vi "CtrlFindHandler.vi"(3 "Type":T1=enum."Value Change", 4 "Ctrl":refnum<vi>, 5 "Structure":refnum<vi>) -> (0 "Index":i32, 1 "Frame":i32, 2 "Diagram":refnum<vi>)   [LabVIEW 2014]
uses:
  <vilib>/event_ctls.llb/lveventtype.ctl
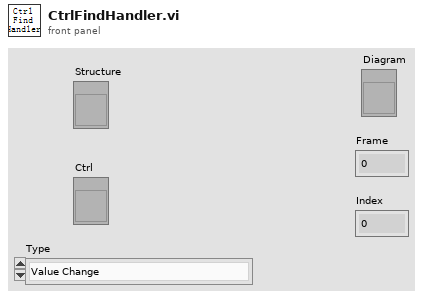
[diagram p1: front panel]
types:
  T1 = typedef "lveventtype.ctl" = enum32{"Null", "Timeout", "Annotation Menu Selection", "Annotation Menu Selection?", "App Instance Close", "App Instance Close?", "Autoscale Range Change", "Bookmark Info Change", "Cell Edit", "Cell Edit?", "Cursor Grab", "Cursor Grab?", "Cursor Menu Selection", "Cursor Menu Selection?", "Cursor Move", "Cursor Release", "Data Change", "Direction Change", "Display State Change", "Drag Ended", "Drag Enter", "Drag Leave", "Drag Over", "Drag Source Update", "Drag Starting", "Drag Starting?", "Drop", "Exec State Change", "Key Down", "Key Down?", "Key Repeat", "Key Repeat?", "Key Up", "Listbox Double Click", "Menu Activation?", "Menu Selection (App)", "Menu Selection? (App)", "Menu Selection (User)", "Mouse Down", "Mouse Down?", "Mouse Enter", "Mouse Leave", "Mouse Move", "Mouse Up", "Mouse Wheel", "NI Security User Change (App)", "Pane Size", "Panel Close", "Panel Close?", "Panel Resize", "Plot Attribute Change", "Scale Range Change", "Shortcut Menu Activation?", "Shortcut Menu Selection (App)", "Shortcut Menu Selection? (App)", "Shortcut Menu Selection (User)", "Tree Double Click", "Tree Drag", "Tree Drag?", "Tree Drop", "Tree Drop?", "Tree Item Close", "Tree Item Close?", "Tree Item Open", "Tree Item Open?", "User Event", "Value Change"}
  T2 = cluster{"Event Type":T1, "Reference":refnum<vi>, "Limit (-1=none)":i32, "Lock Panel?":bool}[]
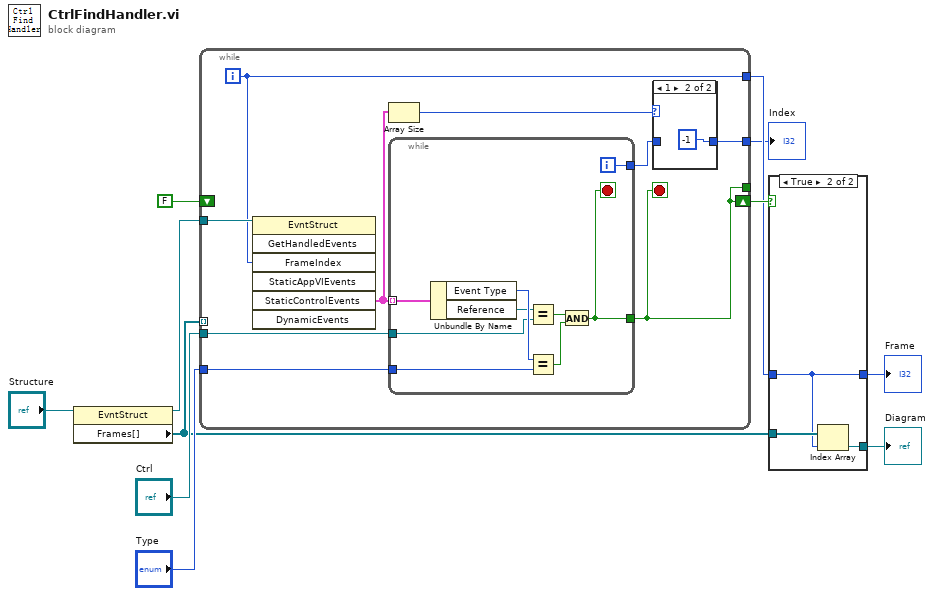
[diagram p0: block diagram]
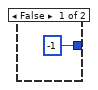
[diagram p2: hidden frame]
diagram:
  n1 = property class="EvntStruct"(reference="Structure") -> (reference out=w10:refnum<vi>, "Frames[]"=w2:refnum<vi>[])  [unwired: 1 in, 1 out]
  n2 = while {
    tunnel: "Type" -> [w20]
    tunnel: "Ctrl" -> [w19]
    tunnel: w10 -> [w18]
    tunnel: [w17] -> w5
    shift-right: [w16] -> w6
    shift-left: FALSE -> [_]
    tunnel: w2 -> [_] mode=indexing
    tunnel: [w16] -> _
    tunnel: [w12] -> w3
    i -> [w17]
    stop <- w16 stop-if-true
    n3 = invoke class="EvntStruct" method="GetHandledEvents"(reference=w18, "FrameIndex"=w17) -> ("StaticControlEvents"=w15:T2)  [unwired: 5 in, 6 out]
    n4 = Array Size(array=w15) -> (size(s)=w14:i32)
    n5 = while {
      tunnel: w15 -> [w31] mode=indexing
      tunnel: w20 -> [w29]
      tunnel: w19 -> [w27]
      tunnel: [w24] -> w16
      tunnel: [w23] -> w13
      i -> [w23]
      stop <- w24 stop-if-true
      n6 = Unbundle By Name(w31) -> ("Event Type"=w30:T1, "Reference"=w28:refnum<vi>)
      n7 = Equal?(x=w28, y=w27) -> (x = y?=w26:bool)
      n8 = Equal?(x=w30, y=w29) -> (x = y?=w25:bool)
      n9 = And(x=w26, y=w25) -> (x .and. y?=w24:bool)
    }
    n10 = case shown="1" w14 {
      tunnel: w13 -> [w21 _]
      tunnel: [w21 -1] -> w12
      frame Default {
      }
      frame 1 {
      }
    }
  }
  "Index" <- w3
  n11 = case shown="True" w6 {
    tunnel: w5 -> [_ w34]
    tunnel: [-1 w34] -> w4
    tunnel: w2 -> [_ w35]
    tunnel: [_ w33] -> w1
    frame False {
    }
    frame True {
      n12 = Index Array(array=w35, index=w34) -> (element=w33:refnum<vi>)
    }
  }
  "Frame" <- w4
  "Diagram" <- w1
